vi "Debug - Flatten Dtacq Connection to Strings.vi"(11 "DTACQ Connection Data In":T1) -> (2 "Array of Strings":string[](array[string]))   [LabVIEW 2017, in "Communications Library.lvlib"]
doc: "Creates an array of strings describing the DTACQ TCP connection details.\n\nUse to create debug logs."
uses:
  Communications Library.lvlib
  Typedefs/DTACQ Connection Data--Cluster.ctl
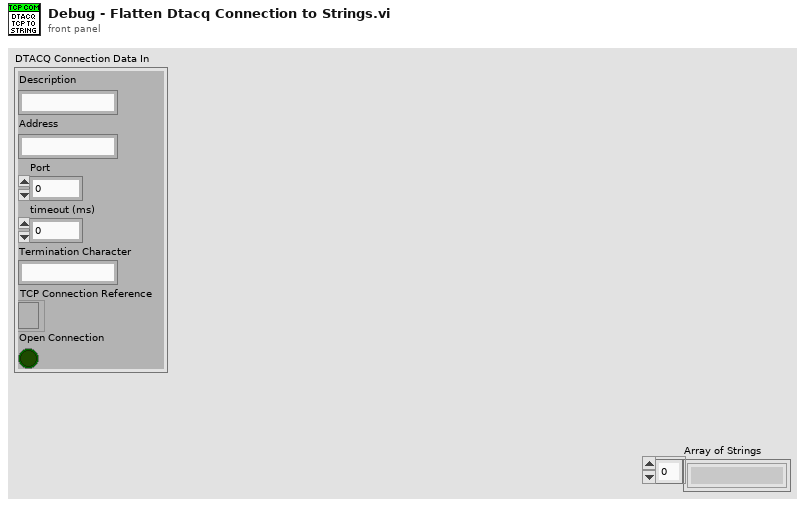
[diagram p1: front panel]
types:
  T1 = typedef "Communications Library.lvlib/DTACQ Connection Data--Cluster.ctl" = cluster{"Description":string, "Address":string, "Port":u16, "timeout (ms)":i32, "Termination Character":string, "TCP Connection Reference":refnum<k5>, "Open Connection":bool}
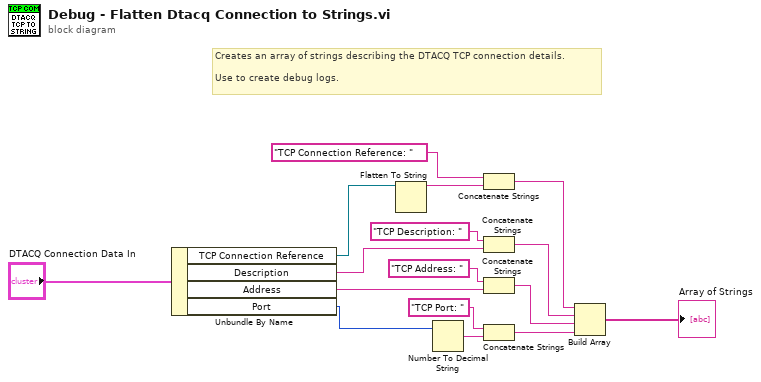
[diagram p0: block diagram]
diagram:
  # "Creates an array of strings describing the DTACQ TCP connection details.\n\nUse to create debug logs."
  n1 = Unbundle By Name("DTACQ Connection Data In") -> ("TCP Connection Reference"=w5:refnum<k5>, "Description"=w11:string, "Address"=w9:string, "Port"=w2:u16)
  n2 = Flatten To String(anything=w5) -> (data string=w6:string)  [unwired: 3 in, 2 out]
  n3 = Number To Decimal String(number=w2) -> (decimal integer string=w3:string)  [unwired: 1 in]
  n4 = Concatenate Strings("TCP Connection Reference: " ("string"), w6) -> (w13:string)
  n5 = Concatenate Strings("TCP Description: " ("string"), w11) -> (w14:string)
  n6 = Concatenate Strings("TCP Address: " ("string"), w9) -> (w15:string)
  n7 = Concatenate Strings("TCP Port: " ("string"), w3) -> (w12:string)
  n8 = Build Array(w13, w14, w15, w12) -> (→"Array of Strings":string[])
